vi "DMA.Configure (Block).vi"(7 "Transfer Direction":enum16{"Write", "Read"}(ring), 8 "error in (no error)":errorcluster, 10 "Block Transfer Spec":T1 {"Block Descriptor"."next descriptor ptr" format="%08x"; "Block Descriptor"."data size" format="%08x"; "Block Descriptor"."data ptr (upper)" format="%08x"; "Block Descriptor"."data ptr (lower)" format="%08x"; "Block Descriptor"."descriptor ptr (aligned)" format="%08x"; "Block Descriptor"."descriptor size" format="%08x"; "Block Descriptor"."descriptor ptr (VISA)" format="%08x"; "RFM Address" format="%08x"}, 11 "GE 5565PIORC":refnum<class "GE 5565PIORC.lvclass">) -> (0 "error out":errorcluster, 3 "GE 5565PIORC out":refnum<class "GE 5565PIORC.lvclass">)   [LabVIEW 2016, in "GE 5565PIORC.lvclass"]
uses:
  GE 5565PIORC.lvclass
  Controls/DMA Transfer Spec (Block).ctl
  Controls/DMA Block Descriptor.ctl
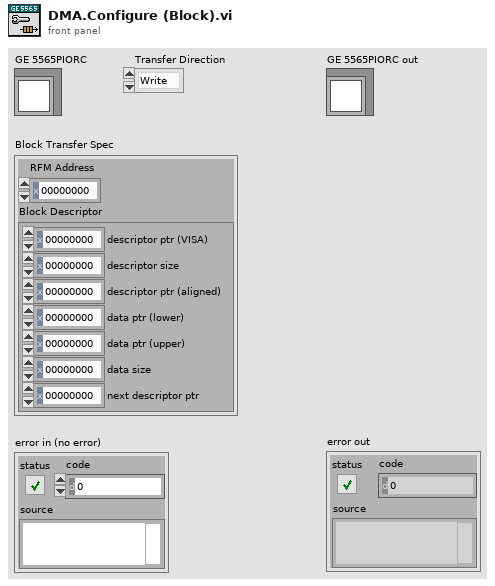
[diagram p1: front panel]
types:
  T1 = typedef "GE 5565PIORC.lvclass/DMA Transfer Spec (Block).ctl" = cluster{"RFM Address":u32, "Block Descriptor":T2}
  T2 = typedef "GE 5565PIORC.lvclass/DMA Block Descriptor.ctl" = cluster{"descriptor ptr (VISA)":u32, "descriptor size":u32, "descriptor ptr (aligned)":u32, "data ptr (lower)":u32, "data ptr (upper)":u32, "data size":u32, "next descriptor ptr":u32}
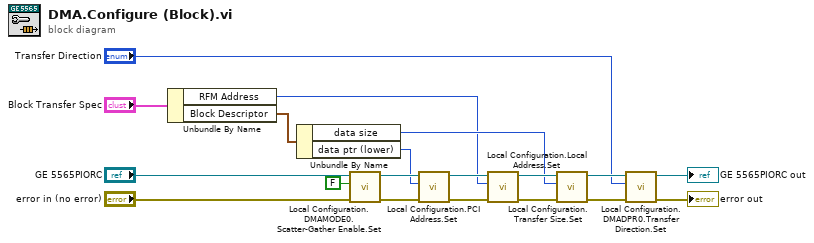
[diagram p0: block diagram]
diagram:
  n1 = Unbundle By Name("Block Transfer Spec") -> ("RFM Address"=w2:u32, "Block Descriptor"=w19:T2)
  n2 = Unbundle By Name(w19) -> ("data size"=w3:u32, "data ptr (lower)"=w1:u32)
  n3 = call "Local Configuration.DMAMODE0.Scatter-Gather Enable.Set.vi"("error in (no error)"="error in (no error)", "Enable Scatter-Gather DMA?"=FALSE, "GE 5565PIORC"="GE 5565PIORC") -> ("error out"=w14:errorcluster, "GE 5565PIORC out"=w8:refnum<class "GE 5565PIORC.lvclass">)  [unwired: 7 in]
  n4 = call "Local Configuration.PCI Address.Set.vi"("error in (no error)"=w14, "PCI Address"=w1, "GE 5565PIORC"=w8) -> ("error out"=w13:errorcluster, "GE 5565PIORC out"=w7:refnum<class "GE 5565PIORC.lvclass">)  [unwired: 7 in]
  n5 = call "Local Configuration.Local Address.Set.vi"("error in (no error)"=w13, "Local Address"=w2, "GE 5565PIORC"=w7) -> ("error out"=w12:errorcluster, "GE 5565PIORC out"=w6:refnum<class "GE 5565PIORC.lvclass">)  [unwired: 7 in]
  n6 = call "Local Configuration.Transfer Size.Set.vi"("error in (no error)"=w12, "Transfer Size"=w3, "GE 5565PIORC"=w6) -> ("error out"=w11:errorcluster, "GE 5565PIORC out"=w5:refnum<class "GE 5565PIORC.lvclass">)  [unwired: 7 in]
  n7 = call "Local Configuration.DMADPR0.Transfer Direction.Set.vi"("error in (no error)"=w11, "Transfer Direction"="Transfer Direction", "GE 5565PIORC"=w5) -> ("error out"=→"error out":errorcluster, "GE 5565PIORC out"=→"GE 5565PIORC out":refnum<class "GE 5565PIORC.lvclass">)  [unwired: 7 in]
